vi "Rebin Plot with Dialog.vi"(8 "error in (no error)":errorcluster, 11 "Original Bin Histogram":cluster{"Axis":dbl[], "Histogram":dbl[]}) -> (0 "error out":errorcluster, 1 "Binning Factor_":dbl format="%#g", 2 "Bin Size_":dbl caption="Bin Size" format="%#g", 3 "Rebinned Histogram":cluster{"Axis":dbl[], "Histogram":dbl[]}, 4 "OK?":bool)   [LabVIEW 2021, in "Histogram Window.lvlib"]
uses:
  Histogram Window.lvlib
  <userlib>/_OpenG.lib/array/array.llb/Filter 1D Array with Scalar (DBL)__ogtk.vi
  <userlib>/_OpenG.lib/array/array.llb/openg_array.lvlib
  c11c0305-7e35-4939-96b6-cedb7b6ff26b.vi
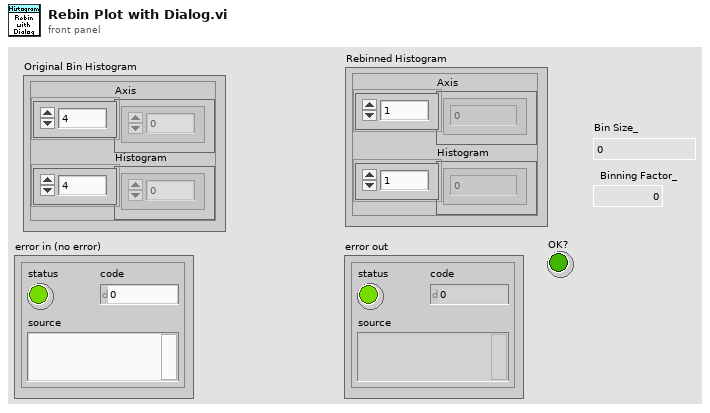
[diagram p1: front panel]
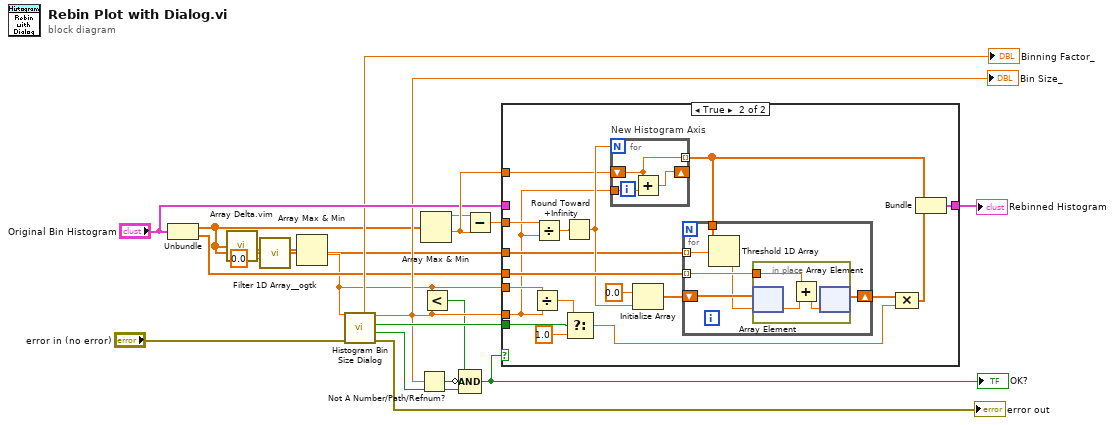
[diagram p0: block diagram]
diagram:
  n1 = Unbundle("Original Bin Histogram") -> ("Axis"=w1:dbl[], "Histogram"=w6:dbl[])
  n2 = call "Array Delta.vim"("A[i]"=w1) -> ("A[i+1]-A[i]"=w5:dbl[])  [unwired: 8 in]
  n3 = call-poly <userlib>:"Filter 1D Array__ogtk.vi"("items to filter"=0.0, "array"=w5) -> ("filtered array"=w3:dbl[])  [unwired: 4 in, 1 out]
  n4 = Array Max & Min(array=w3) -> (min value=w2:dbl)  [unwired: 3 out]
  n5 = call "Histogram Bin Size Dialog.vi"("error in (no error)"="error in (no error)", "Current Bin Size"=w2) -> ("error out"=→"error out":errorcluster, "OK"=w19:bool, "Rescale Plot_"=w10:bool, "Bin Size_"=w9:dbl, "Binning Factor_"=→"Binning Factor_":dbl)  [unwired: 5 in]
  "Bin Size_" <- w9
  n6 = Not A Number/Path/Refnum?(number/path/refnum=w9) -> (NaN/Path/Refnum?=w11:bool)
  n7 = Array Max & Min(array=w1) -> (max value=w13:dbl, min value=w16:dbl)  [unwired: 2 out]
  n8 = Less?(x=w2, y=w9) -> (x < y?=w8:bool)
  n9 = Compound Arithmetic op=AND(w8, invert w11, w19) -> (w18:bool)
  "OK?" <- w18
  n10 = Subtract(x=w13, y=w16) -> (x-y=w12:dbl)
  n11 = case shown="True" w18 {
    tunnel: w16 -> [_ w34]
    tunnel: w9 -> [_ w27]
    tunnel: w6 -> [_ w37]
    tunnel: w1 -> [_ w33]
    tunnel: [w21 w30] -> w15
    tunnel: "Original Bin Histogram" -> [w21 _]
    tunnel: w12 -> [_ w29]
    tunnel: w10 -> [_ w25]
    tunnel: w2 -> [_ w28]
    frame False {
    }
    frame True {
      n12 = Divide(x=w28, y=w27) -> (x/y=w24:dbl)
      n13 = Divide(x=w29, y=w27) -> (x/y=w39:dbl)
      n14 = Round Toward +Infinity(x=w39) -> (ceil(x): smallest int >= x=w35:dbl)
      n15 = Select(t=w24, s=w25, f=1.0) -> (s? t:f=w22:dbl)
      n16 = for "New Histogram Axis" {
        N: w35 -> [_]
        shift-right: [w41] -> _
        shift-left: w34 -> [w40]
        tunnel: w27 -> [w42]
        tunnel: [w40] -> w32 mode=indexing
        n17 = Add(x=w40, y=w42) -> (x+y=w41:dbl)
      }
      n18 = Initialize Array(0.0 ("element"), w35) -> (w36:dbl[])
      n19 = for {
        tunnel: w37 -> [w46] mode=indexing
        shift-right: [w47] -> w31
        shift-left: w36 -> [w48]
        tunnel: w33 -> [w44] mode=indexing
        tunnel: w32 -> [w45]
        n20 = Threshold 1D Array(2:w44, 3:w45) -> (0:w43:dbl)  [unwired: 1 in]
        n21 = in-place {
          in-place-border: w46 -> [w50]
          n22 = in-place-array #1(w48, w43) -> (w51:dbl)
          n23 = Add(x=w50, y=w51) -> (x+y=w49:dbl)
          n24 = in-place-array #1(w49) -> (w47:dbl[])  [unwired: 1 out]
        }
      }
      n25 = Compound Arithmetic op=MULTIPLY(w31, w22) -> (w26:dbl[])
      n26 = Bundle(w32, w26) -> (w30:cluster{dbl[], dbl[]})  [unwired: 1 in]
    }
  }
  "Rebinned Histogram" <- w15
